vi "EOL CAN_Go to Position.vi"(6 "Postion":u16=3 format="%04x", 7 "Rx Arbitration Id":u32=402522244 format="%.0x", 8 "Error in":errorcluster, 9 "Glass?":bool, 10 "Read Session in":refnum<k21>, 11 "Write Session in":refnum<k21>) -> (0 "Error out":errorcluster, 2 "TxRx Data":string[][](array[string]), 3 "Response Good?":bool)   [LabVIEW 2018]
uses:
  <vilib>/xnet/xnet.llb/XNET Frame CAN.ctl
  <vilib>/xnet/xnet.llb/XNET Frame Type CAN.ctl
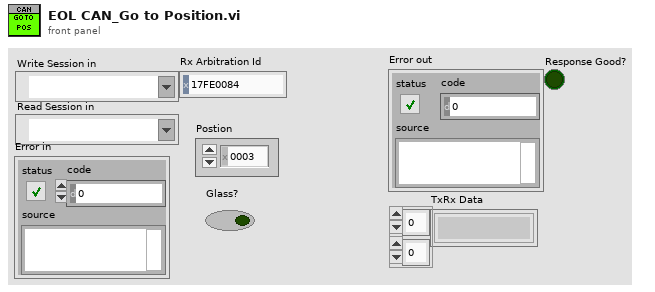
[diagram p1: front panel]
types:
  T1 = typedef "XNET Frame CAN.ctl" = cluster{"timestamp":timestamp, "payload":u8[], "identifier":u32, "type":T2, "extended?":bool, "echo?":bool}
  T2 = typedef "XNET Frame Type CAN.ctl" = u8
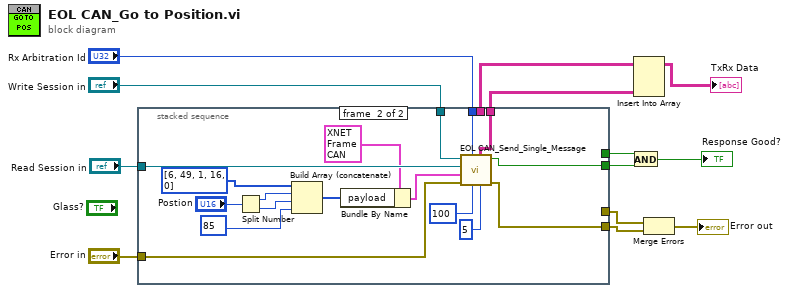
[diagram p0: block diagram]
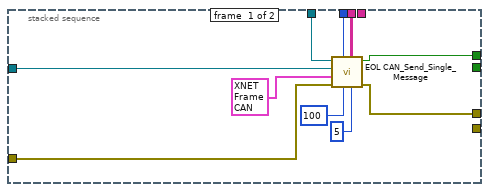
[diagram p2: hidden frame]
diagram:
  n1 = stacked-sequence {
    tunnel: "Error in" -> [w23 w40]
    tunnel: [w22 _] -> w9
    tunnel: "Rx Arbitration Id" -> [w21 w39]
    tunnel: "Write Session in" -> [w20 w38]
    tunnel: "Read Session in" -> [w19 w37]
    tunnel: [w18 _] -> w3
    tunnel: [_ w26] -> w8
    tunnel: [_ w25] -> w2
    tunnel: [w14 _] -> w5
    tunnel: [_ w24] -> w4
    frame #0 {
      n2 = call "EOL CAN_Send_Single_Message.vi"("Retries"=5, "Msg Wait Time"=u32 100, "Rx Arbitration Id"=w21, "Error in"=w23, "Tx CAN frame"=T1 {"timestamp"=timestamp(0 s since 1904-01-01), "payload"=[2, 16, 79, 85, 85, 85, 85, 85], "identifier"=402391172, "type"=8, "extended?"=TRUE, "echo?"=FALSE}, "Read Session in"=w19, "Write Session in"=w20) -> ("Error out"=w14:errorcluster, "Response Good?"=w18:bool, "TxRx Data"=w22:string[][])  [unwired: 2 out]
    }
    frame #1 {
      n3 = Split Number(x="Postion") -> (hi(x)=w30:u8, lo(x)=w31:u8)
      n4 = Build Array (concatenate)(u8[] [6, 49, 1, 16, 0] ("payload"), w30, w31, u8 85 ("Numeric")) -> (w34:u8[])
      n5 = Bundle By Name(cluster=T1 {"timestamp"=timestamp(0 s since 1904-01-01), "payload"=[3, 34, 241, 134, 85, 85, 85, 85], "identifier"=402391172, "type"=8, "extended?"=TRUE, "echo?"=FALSE} ("CAN frame"), "payload"=w34) -> (w27:T1)
      n6 = call "EOL CAN_Send_Single_Message.vi"("Retries"=5, "Msg Wait Time"=u32 100, "Rx Arbitration Id"=w39, "Error in"=w40, "Tx CAN frame"=w27, "Read Session in"=w37, "Write Session in"=w38) -> ("Error out"=w24:errorcluster, "Response Good?"=w25:bool, "TxRx Data"=w26:string[][])  [unwired: 2 out]
    }
  }
  n7 = And(x=w3, y=w2) -> (x .and. y?=→"Response Good?":bool)
  n8 = Insert Into Array(array=w9, new element=w8) -> (→"TxRx Data":string[][])  [unwired: 2 in]
  n9 = Merge Errors(w5, w4) -> (→"Error out":errorcluster)
